vi "Get Strings from Ref.vi"(8 "error in (no error)":errorcluster, 9 "Label Prefix":string, 10 "GObj Refnum in":refnum<vi>, 11 "RingControl in":refnum<class "TabControl.lvclass">) -> (0 "error out":errorcluster, 1 "Valid?":bool, 2 "GObj Refnum out":refnum<vi>, 3 "RingControl out":refnum<class "TabControl.lvclass">, 4 "GObj Name":string)   [LabVIEW 2013, in "SET Project Data.lvlib" / "TabControl.lvclass"]
uses:
  TabControl.lvclass
  Control/Control.lvclass
  GObject/GObject.lvclass/GObject.ctl
  GObject/Write UID.vi
  SET Project Data.lvlib
  GObject/GObject.lvclass
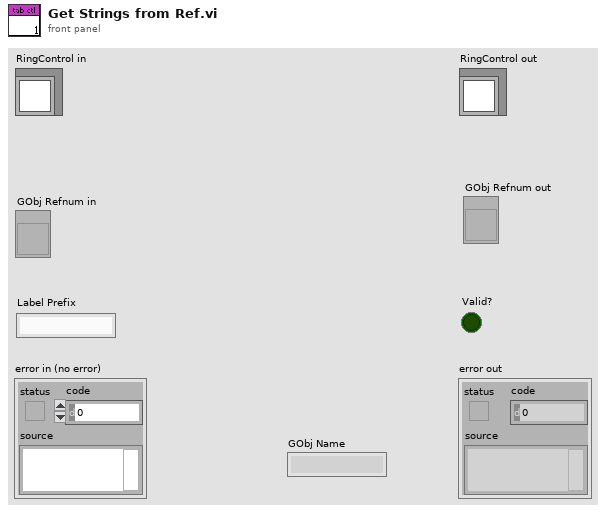
[diagram p1: front panel]
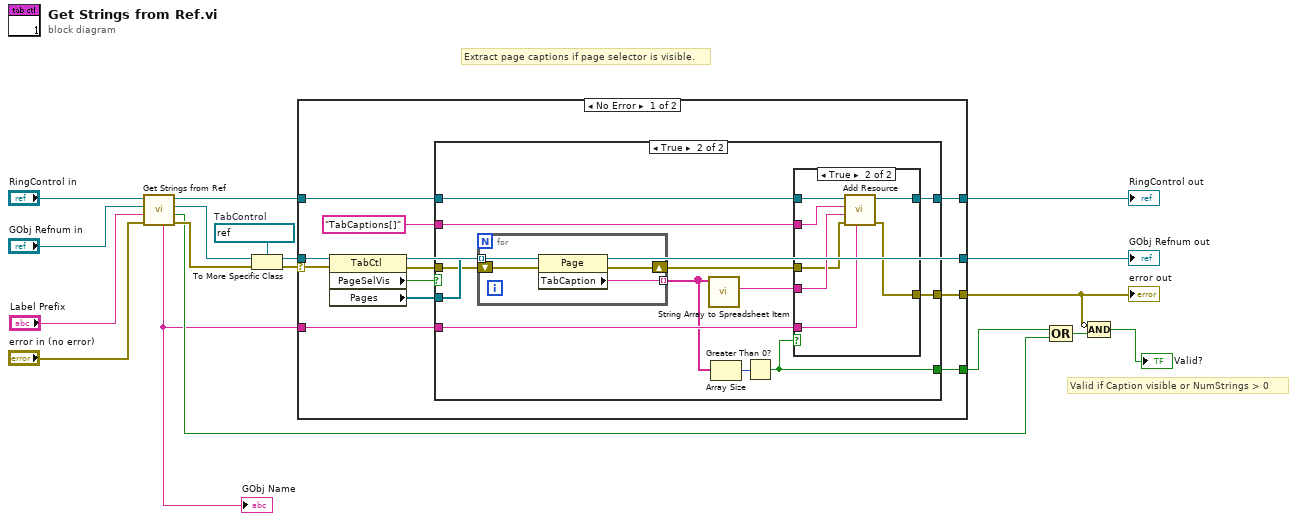
[diagram p0: block diagram]
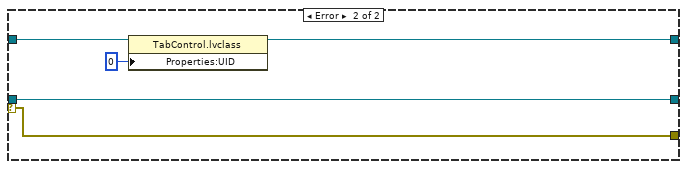
[diagram p4: hidden frame]
diagram:
  w13 = refnum<vi> refnum  # TabControl
  # "Extract page captions if page selector is visible."
  # "Valid if Caption visible or NumStrings > 0"
  n1 = call-parent "Get Strings from Ref.vi"("error in (no error)"="error in (no error)", "Label Prefix"="Label Prefix", "GObj Refnum in"="GObj Refnum in", "Control in"="RingControl in") -> ("error out"=w14:errorcluster, "Valid?"=w6:bool, "GObj Refnum out"=w15:refnum<vi>, "Control out"=w10:refnum<class "TabControl.lvclass">, "GObj Name"=w1:string)  [unwired: 3 in]
  "GObj Name" <- w1
  n2 = To More Specific Class(target class=w13, reference=w15, error in=w14) -> (specific class reference=w12:refnum<vi>, error out=w11:errorcluster)
  n3 = case shown="No Error" w11 {
    selector: w11 -> [w29 w61]
    tunnel: w12 -> [w30 w62]
    tunnel: w10 -> [w28 w60]
    tunnel: [w27 w58] -> w9
    tunnel: [w24 w61] -> w4
    tunnel: [w19 w62] -> w8
    tunnel: [w23 _] -> w7
    tunnel: w1 -> [w22 _]
    frame No Error {
      n4 = property class="TabCtl"(reference=w30, error in=w29) -> (reference out=w19:refnum<vi>, error out=w25:errorcluster, "PageSelVis"=w21:bool, "Pages"=w20:refnum<vi>[])
      n5 = case shown="True" w21 {
        tunnel: w28 -> [w32 w43]
        tunnel: [w32 w42] -> w27
        tunnel: "TabCaptions[]" -> [_ w40]
        tunnel: w25 -> [w31 w35]
        tunnel: [w31 w39] -> w24
        tunnel: [_ w38] -> w23
        tunnel: w22 -> [_ w37]
        tunnel: w20 -> [_ w36]
        frame False {
        }
        frame True {
          n6 = for {
            tunnel: w36 -> [w48] mode=indexing
            shift-right: [w46] -> w33
            shift-left: w35 -> [w47]
            tunnel: [w45] -> w34 mode=indexing
            n7 = property class="Page"(reference=w48, error in=w47) -> (error out=w46:errorcluster, "TabCaption"=w45:string)  [unwired: 1 out]
          }
          n8 = call "String Array to Spreadsheet Item.vi"("Strings [] (ASCII)"=w34) -> ("Spreadsheet Item (ASCII)"=w41:string)  [unwired: 10 in]
          n9 = Array Size(array=w34) -> (size(s)=w44:i32)
          n10 = Greater Than 0?(x=w44) -> (x > 0?=w38:bool)
          n11 = case shown="True" w38 {
            tunnel: w43 -> [w50 w57]
            tunnel: [w50 w56] -> w42
            tunnel: w37 -> [_ w55]
            tunnel: w41 -> [_ w54]
            tunnel: w40 -> [_ w53]
            tunnel: w33 -> [w49 w52]
            tunnel: [w49 w51] -> w39
            frame False {
            }
            frame True {
              n12 = call "Add Resource.vi"("TagPrefix"=w55, "error in (no error)"=w52, "ItemText"=w54, "ItemName"=w53, "GObject in"=w57) -> ("error out"=w51:errorcluster, "GObject out"=w56:refnum<class "TabControl.lvclass">)  [unwired: 5 in]
            }
          }
        }
      }
    }
    frame Error {
      n13 = property class="TabControl.lvclass"(reference=w60, "Properties:UID"=0 ("UID")) -> (reference out=w58:refnum<class "TabControl.lvclass">)  [unwired: 1 in, 1 out]
    }
  }
  "error out" <- w4
  "RingControl out" <- w9
  "GObj Refnum out" <- w8
  n14 = Compound Arithmetic op=OR(w7, w6) -> (w5:bool)
  n15 = Compound Arithmetic op=AND(invert w4, w5) -> (→"Valid?":bool)
